vi "Write Configuration File.vi"(11 "error in (no error)":errorcluster) -> (15 "error out":errorcluster)   [LabVIEW 2014]
uses:
  <vilib>/Utility/config.llb/NI_LVConfig.lvlib
panel:
  in  "Config File Path":path
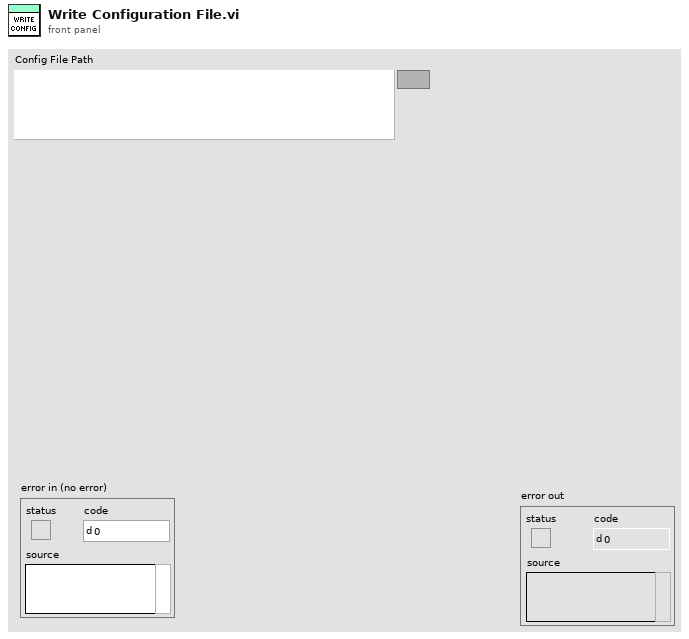
[diagram p1: front panel]
types:
  T1 = typedef "NI_LVConfig.lvlib/Config Data RefNum.ctl" = refnum<k1>
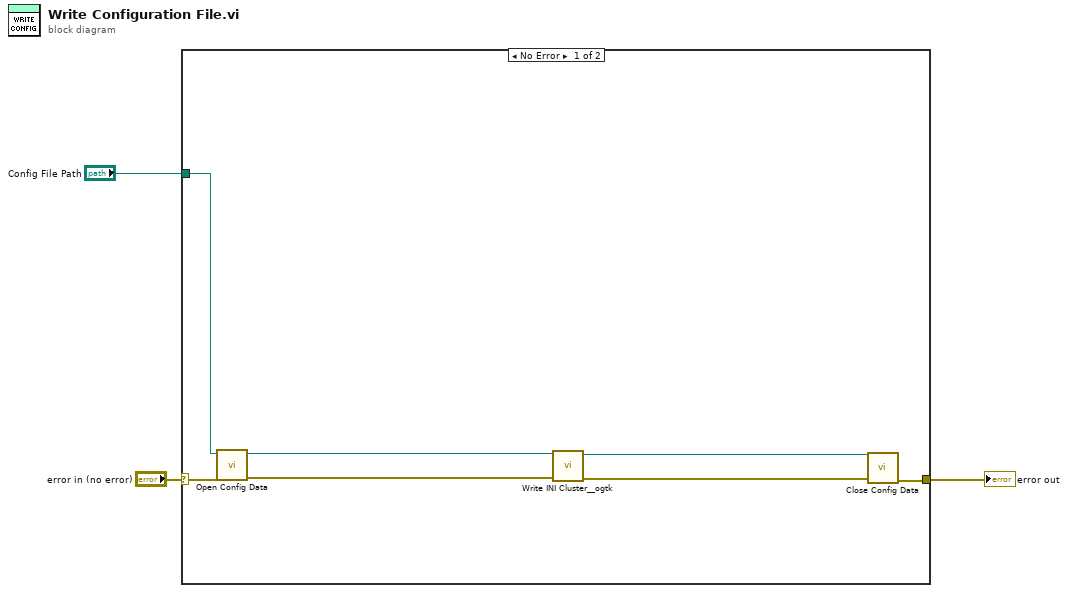
[diagram p0: block diagram]
diagram:
  n1 = case shown="No Error" "error in (no error)" {
    selector: "error in (no error)" -> [w10 w11]
    tunnel: [w8 w11] -> w2
    tunnel: "Config File Path" -> [w9 _]
    frame No Error {
      n2 = call <vilib>:"Open Config Data.vi"("error in (no error)"=w10, "configuration file path"=w9) -> ("error out"=w7:errorcluster, "refnum"=w5:T1)  [unwired: 7 in, 1 out]
      n3 = call <userlib>:"Write INI Cluster__ogtk.vi"("error in (no error)"=w7, "refnum"=w5) -> ("error out"=w6:errorcluster, "dup refnum"=w4:T1)  [unwired: 8 in]
      n4 = call <vilib>:"Close Config Data.vi"("error in (no error)"=w6, "refnum"=w4) -> ("error out"=w8:errorcluster)  [unwired: 8 in, 1 out]
    }
    frame Error {
    }
  }
  "error out" <- w2
